vi "wrong_pass.vi"() -> ()   [LabVIEW 2015]
panel:
  in  "OK Button":bool
  # "Password Incorrecto!\nVuelva a intentar"
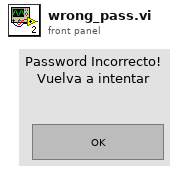
[diagram p1: front panel]
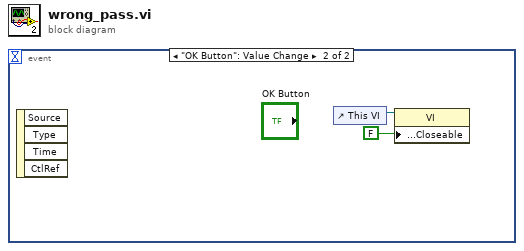
[diagram p0: block diagram]
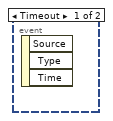
[diagram p2: hidden frame]
diagram:
  n1 = event shown="[1] \"OK Button\": Value Change" {
    selector: _ -> [_ _]
    dyn-events: _ -> [_ _]
    timeout: _ -> [_ _]
    event Timeout {
      n2 = event-data() -> ()  [unwired: 1 in, 3 out]
    }
    event "OK Button": Value Change {
      n3 = event-data() -> ()  [unwired: 1 in, 4 out]
      n4 = control-ref of="This VI"() -> (w2:refnum<vi>)
      n5 = property class="VI"(reference=w2, "Front Panel.Closeable"=FALSE ("Front Panel Window:Closeable")) -> ()  [unwired: 1 in, 2 out]
    }
  }
